vi "Error Query.vi"(6 "error in (no error)":errorcluster, 9 "VISA Resource Name":refnum<visa-resource-name>) -> (0 "error out":errorcluster, 1 "Error Message":string, 2 "Error":i32, 3 "dup VISA session":refnum<visa-resource-name>)   [LabVIEW 2018, in "PNA-X.lvlib"]
uses:
  PNA-X.lvlib
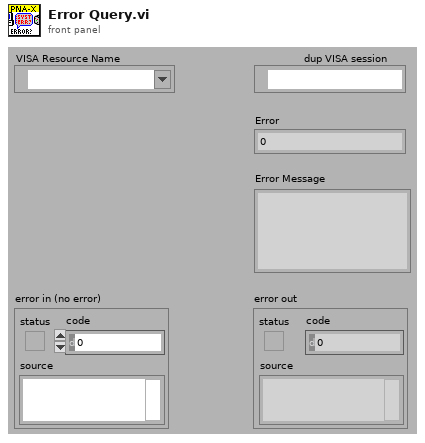
[diagram p1: front panel]
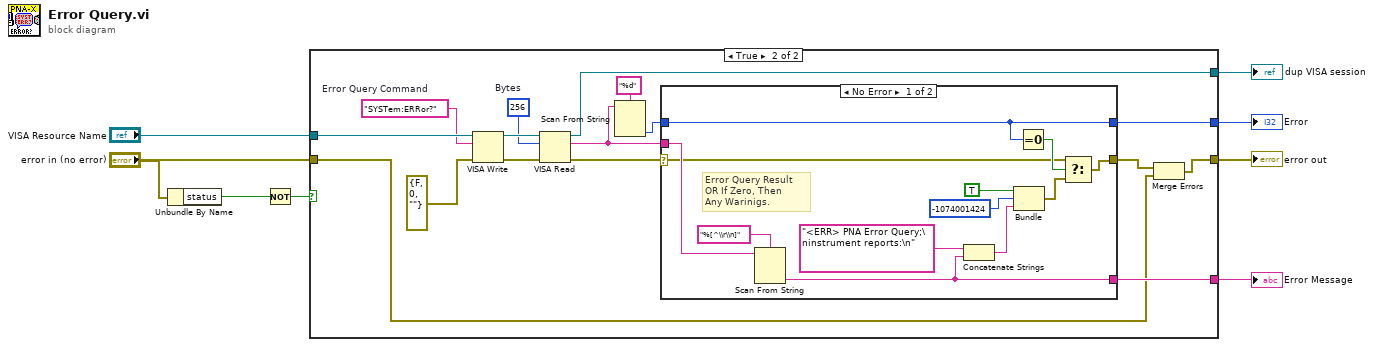
[diagram p0: block diagram]
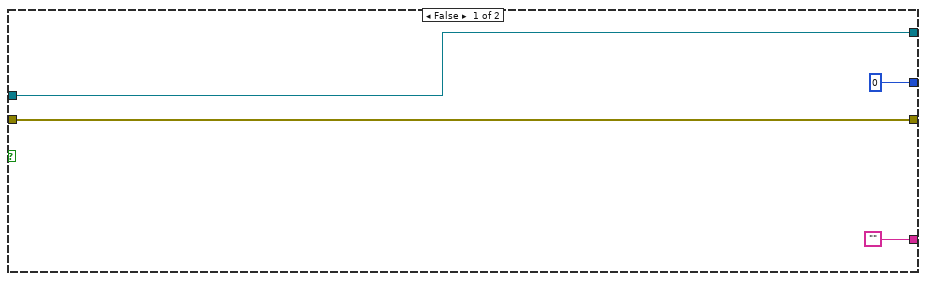
[diagram p2: hidden frame]
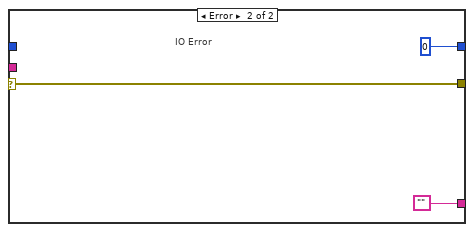
[diagram p3: hidden frame]
diagram:
  n1 = Unbundle By Name("error in (no error)") -> ("status"=w1:bool)
  n2 = Not(x=w1) -> (.not. x?=w2:bool)
  n3 = case shown="True" w2 {
    tunnel: ["" w28] -> w5
    tunnel: [0 w27] -> w4
    tunnel: [w12 w26] -> w3
    tunnel: "VISA Resource Name" -> [w12 w25]
    tunnel: "error in (no error)" -> [w9 w18]
    tunnel: [w9 w17] -> w6
    frame False {
    }
    frame True {
      w23 = u32 256  # Bytes
      w21 = "SYSTem:ERRor?"  # Error Query Command
      n4 = VISA Write(VISA resource name=w25, write buffer=w21, error in (no error)=errorcluster {"status"=FALSE, "code"=0, "source"=""}) -> (VISA resource name out=w24:refnum<visa-resource-name>, error out=w22:errorcluster)  [unwired: 1 out]
      n5 = VISA Read(VISA resource name=w24, byte count=w23, error in (no error)=w22) -> (VISA resource name out=w26:refnum<visa-resource-name>, read buffer=w16:string, error out=w13:errorcluster)  [unwired: 1 out]
      n6 = Scan From String(format string="%d", input string=w16) -> (output 1=w14:i32)  [unwired: 3 in, 3 out]
      n7 = case shown="No Error" w13 {
        selector: w13 -> [w29 w41]
        tunnel: w16 -> [w31 _]
        tunnel: [w36 w41] -> w19
        tunnel: [w32 ""] -> w28
        tunnel: [w30 0] -> w27
        tunnel: w14 -> [w30 _]
        frame No Error {
          # "Error Query Result\nOR If Zero, Then\nAny Warinigs."
          n8 = Scan From String(format string="%[^\\r\\n]", input string=w31) -> (output 1=w32:string)  [unwired: 3 in, 3 out]
          n9 = Concatenate Strings("<ERR> PNA Error Query;\ninstrument reports:\n" ("Source"), w32) -> (w38:string)
          n10 = Bundle("Status"=TRUE, "Code"=-1074001424, w38) -> (w37:cluster{"Status":bool, "Code":i32, string})  [unwired: 1 in]
          n11 = Equal To 0?(x=w30) -> (x = 0?=w34:bool)
          n12 = Select(t=w29, s=w34, f=w37) -> (s? t:f=w36:errorcluster)
        }
        frame Error {
          # "IO Error"
        }
      }
      n13 = Merge Errors(w19, w18) -> (w17:errorcluster)
    }
  }
  "Error Message" <- w5
  "error out" <- w6
  "Error" <- w4
  "dup VISA session" <- w3
